vi "Read.vi"(8 "error in (no error)":errorcluster, 11 "SoftmotionAxis in":refnum<class "SoftmotionAxis.lvclass">) -> (0 "error out":errorcluster, 2 "appended array":dbl[](array[numeric]), 3 "SoftmotionAxis out":refnum<class "SoftmotionAxis.lvclass">)   [LabVIEW 2017, in "SoftmotionAxis.lvclass"]
uses:
  SoftmotionAxis.lvclass
  <resource>/objmgr/nimcai.rc
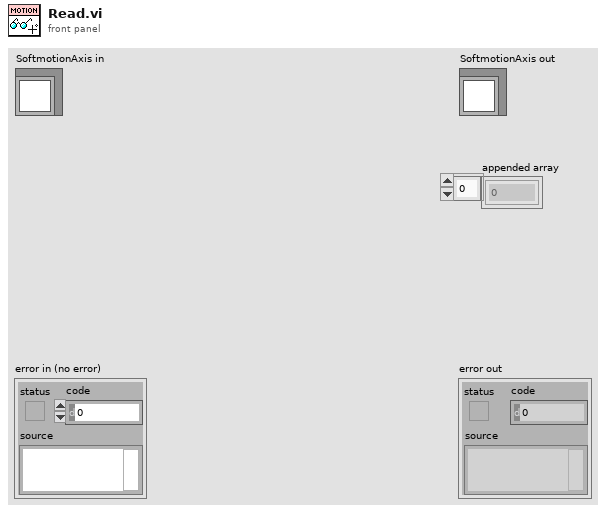
[diagram p1: front panel]
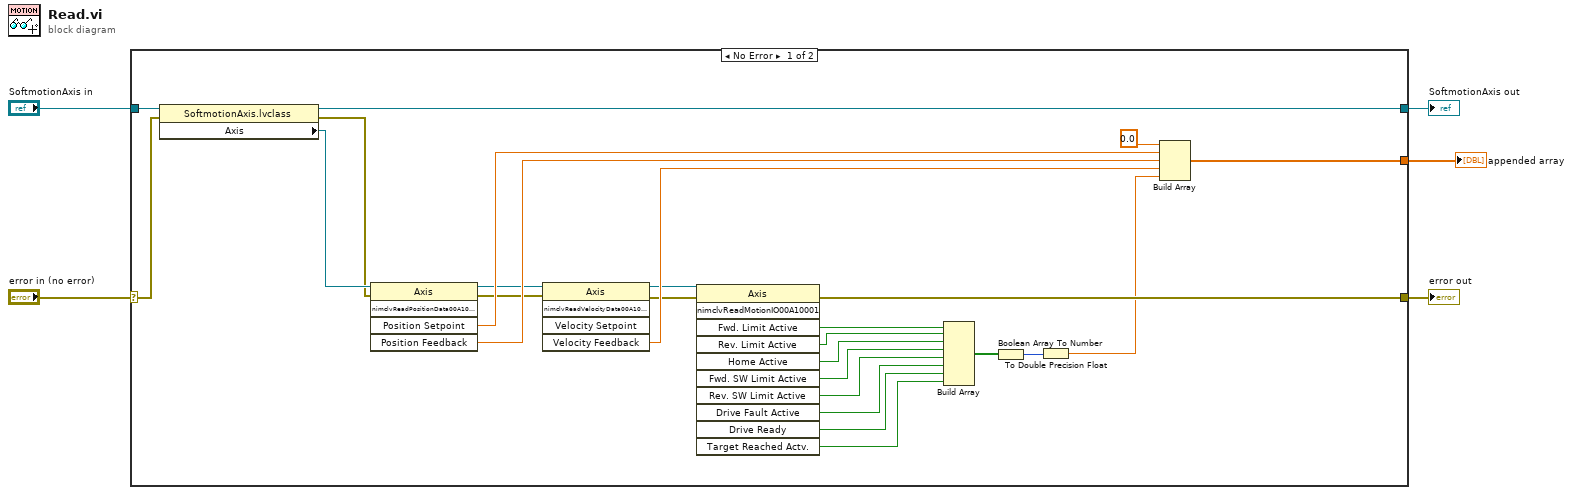
[diagram p0: block diagram]
diagram:
  n1 = case shown="No Error" "error in (no error)" {
    selector: "error in (no error)" -> [w20 w33]
    tunnel: [w19 w33] -> w4
    tunnel: [w17 w32] -> w2
    tunnel: "SoftmotionAxis in" -> [w18 w32]
    tunnel: [w21 _] -> w1
    frame No Error {
      n2 = property class="SoftmotionAxis.lvclass"(reference=w18, error in=w20) -> (reference out=w17:refnum<class "SoftmotionAxis.lvclass">, error out=w10:errorcluster, "Axis"=w11:refnum<k21>)
      n3 = invoke class="Axis" method="nimclvReadPositionData00A10001"(reference=w11, error in=w10) -> (reference out=w9:refnum<k21>, error out=w8:errorcluster, "Position Setpoint"=w15:dbl, "Position Feedback"=w14:dbl)  [unwired: 3 in, 1 out]
      n4 = invoke class="Axis" method="nimclvReadVelocityData00A10001"(reference=w9, error in=w8) -> (reference out=w7:refnum<k21>, error out=w6:errorcluster, "Velocity Feedback"=w13:dbl)  [unwired: 3 in, 2 out]
      n5 = invoke class="Axis" method="nimclvReadMotionIO00A10001"(reference=w7, error in=w6) -> (error out=w19:errorcluster, "Fwd. Limit Active"=w31:bool, "Rev. Limit Active"=w30:bool, "Home Active"=w29:bool, "Fwd. SW Limit Active"=w28:bool, "Rev. SW Limit Active"=w27:bool, "Drive Fault Active"=w26:bool, "Drive Ready"=w25:bool, "Target Reached Actv."=w24:bool)  [unwired: 9 in, 2 out]
      n6 = Build Array(w31, w30, w29, w28, w27, w26, w25, w24) -> (w23:bool[])
      n7 = Boolean Array To Number(Boolean array=w23) -> (number=w22:u32)
      n8 = To Double Precision Float(number=w22) -> (double precision float=w12:dbl)
      n9 = Build Array(0.0 ("element"), w15, w14, w13, w12) -> (w21:dbl[])
    }
    frame Error {
    }
  }
  "error out" <- w4
  "SoftmotionAxis out" <- w2
  "appended array" <- w1
